vi "Setup Waveform Factory.vi"(8 "error in (no error)":errorcluster, 10 "Model in":refnum<class "Model.lvclass">, 11 "Boot Loader in":refnum<class "Boot Loader.lvclass">) -> (0 "error out":errorcluster, 2 "Model out":refnum<class "Model.lvclass">, 3 "Boot Loader out":refnum<class "Boot Loader.lvclass">)   [LabVIEW 2016]
uses:
  Waveforms/Waveform Factory/Waveform Factory.lvclass
  Boot Loader.lvclass
  Model/Model.lvclass
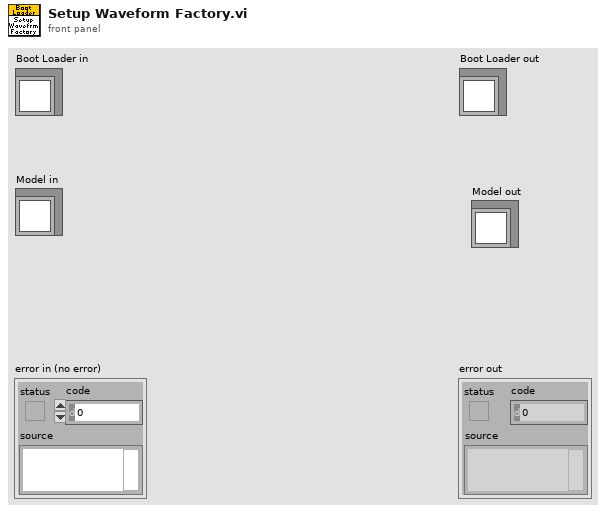
[diagram p1: front panel]
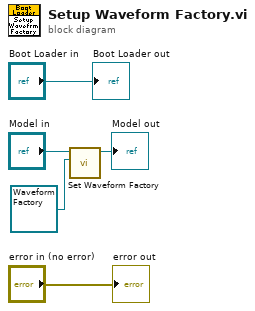
[diagram p0: block diagram]
diagram:
  n1 = call "Set Waveform Factory.vi"("WaveformFactory"=refnum<class "Waveform Factory.lvclass"> refnum ("WaveformFactory.lvclass"), "Model in"="Model in") -> ("Model out"=→"Model out":refnum<class "Model.lvclass">)  [unwired: 9 in]
  "error out" <- "error in (no error)"
  "Boot Loader out" <- "Boot Loader in"
